vi "ws Spartan Uptime.vi"(8 "error in (no error)":errorcluster) -> (0 "error out":errorcluster, 3 "Uptime":dbl)   [LabVIEW 2011]
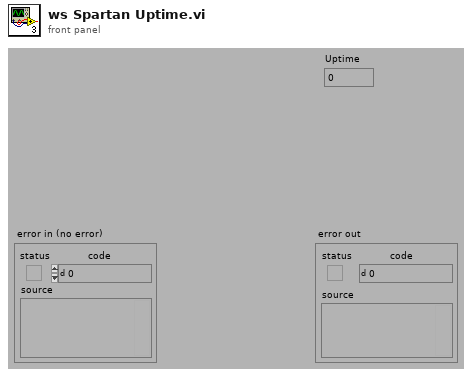
[diagram p1: front panel]
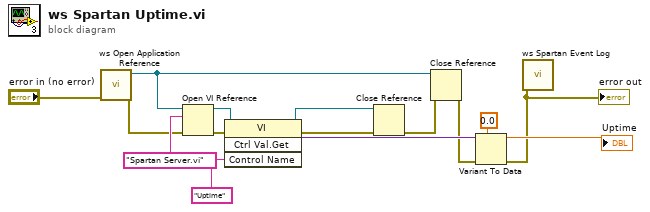
[diagram p0: block diagram]
diagram:
  n1 = call "ws Open Application Reference.vi"("error in (no error)"="error in (no error)") -> ("error out"=w5:errorcluster, "application reference"=w4:refnum<vi>)  [unwired: 9 in]
  n2 = Open VI Reference(application reference (local)=w4, vi path="Spartan Server.vi", error in (no error)=w5) -> (vi reference=w15:refnum<vi>, error out=w14:errorcluster)  [unwired: 3 out]
  n3 = invoke class="VI" method="Ctrl Val.Get"(reference=w15, error in=w14, "Control Name"="Uptime") -> (reference out=w10:refnum<vi>, error out=w3:errorcluster, "Get Control Value Variant"=w12:variant)  [unwired: 1 in, 1 out]
  n4 = Close Reference(reference=w10, error in (no error)=w3) -> (error out=w8:errorcluster)
  n5 = Close Reference(reference=w4, error in (no error)=w8) -> (error out=w2:errorcluster)
  n6 = Variant To Data(error in=w2, type=0.0, Variant=w12) -> (data=→"Uptime":dbl, error out=w1:errorcluster)
  "error out" <- w1
  n7 = call "ws Spartan Event Log.vi"("error in (no error)"=w1) -> ()  [unwired: 7 in, 1 out]
